vi "RX ADU.vi"(8 "error in (no error)":errorcluster, 9 "PDU_req":T1={"Function Code"=1, "Data"=[], "RTU_DataBytes"=0}, 10 "VISA resource in":refnum<visa-resource-name>, 11 "MB_ADU_Serial_ASCII in":refnum<class "MB_ADU_ASCII.lvclass">) -> (0 "error out":errorcluster, 1 "PDU_resp":T1={"Function Code"=1, "Data"=[], "RTU_DataBytes"=0}, 2 "VISA resource out":refnum<visa-resource-name>, 3 "MB_ADU_Serial_ASCII out":refnum<class "MB_ADU_ASCII.lvclass">)   [LabVIEW 2016, in "MB Master.lvlib" / "MB_ADU_ASCII.lvclass"]
doc: "Defines the receive procedure for a Modbus ASCII ADU. The received PDU is written to PDU_resp."
uses:
  MB_ADU_ASCII.lvclass
  C:/Users/illogicdev/Desktop/IGUS/20190906-1xdryveD1+LABview+ModbusTCP(Gateway)/IgusPositioningSystem Folder/Modules/Libraries/Modbus-Master/MB_ADU/MB_ADU.lvclass
  MB_PDU/MB_PDU_Cluster.ctl
  MB_ADU/MB_ADU.lvclass/MB_ADU.ctl
  MB_ADU/Write RX Data.vi
  MB_ADU/Write RX Timestamp.vi
  MB_ADU/Read Slave ID.vi
  MB Master.lvlib
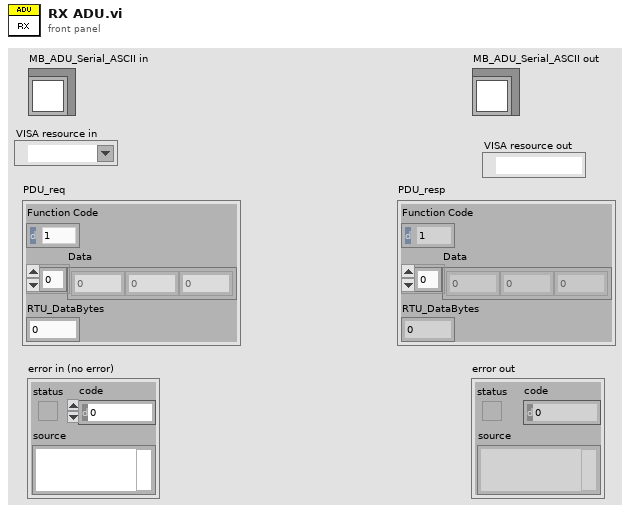
[diagram p1: front panel]
types:
  T1 = typedef "MB Master.lvlib/MB_PDU_Cluster.ctl" = cluster{"Function Code":u8, "Data":u8[], "RTU_DataBytes":i32}
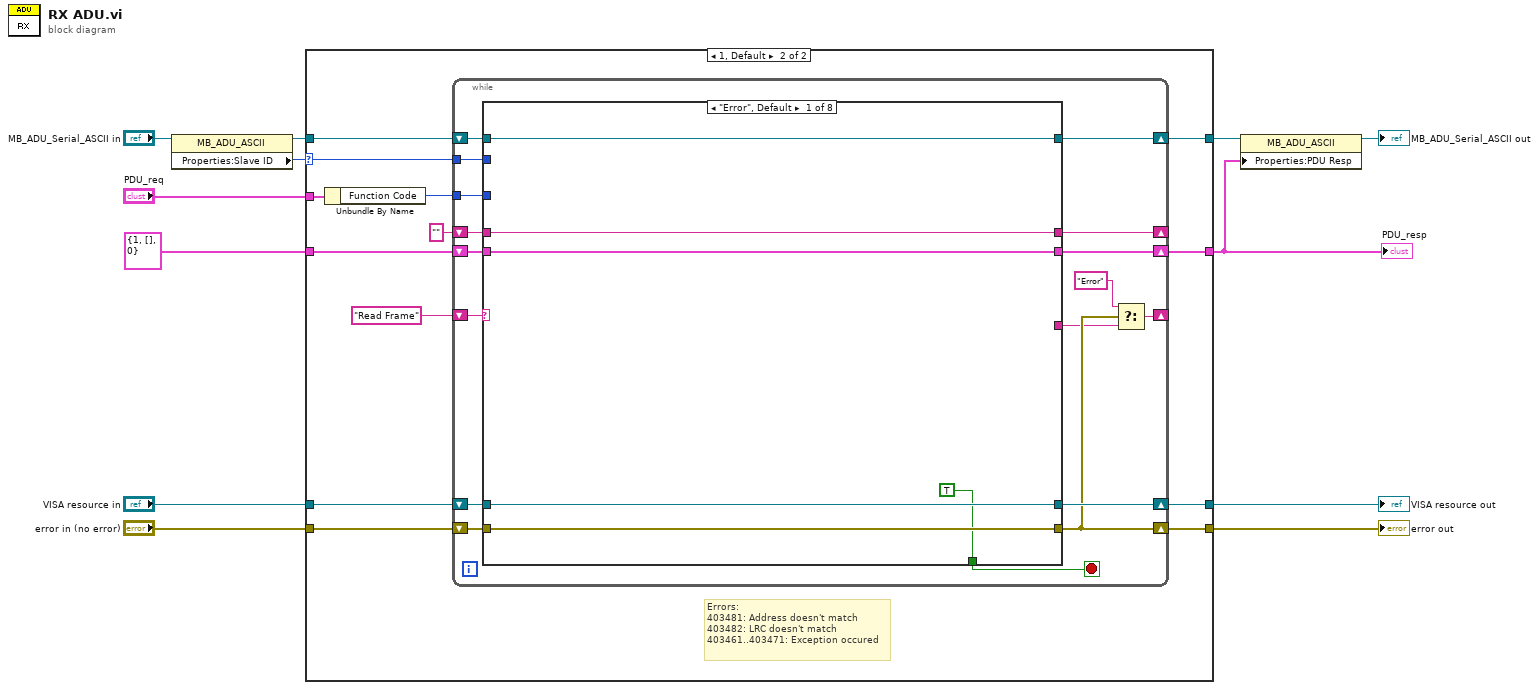
[diagram p0: block diagram]
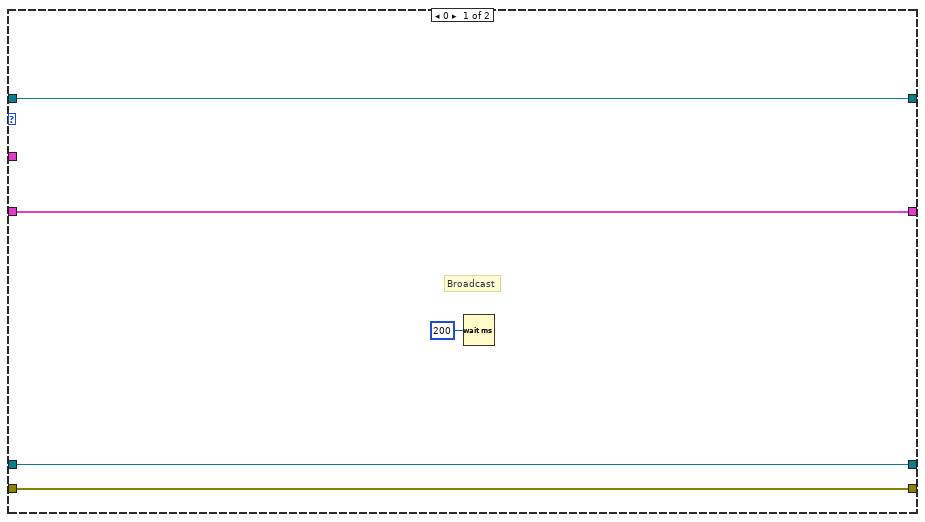
[diagram p2: hidden frame]
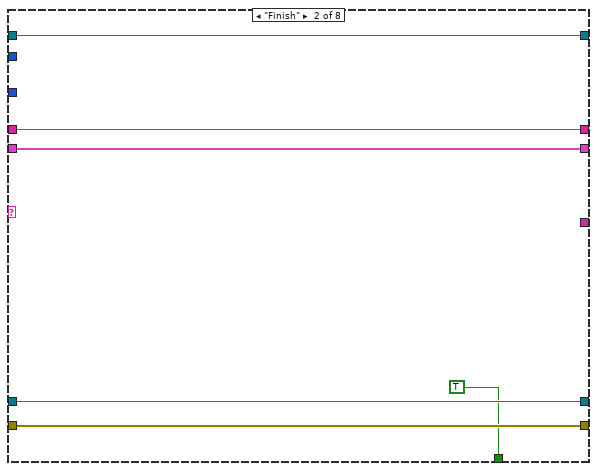
[diagram p3: hidden frame]
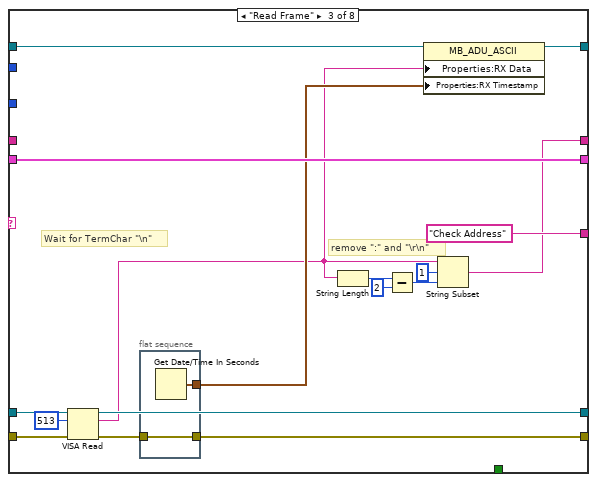
[diagram p4: hidden frame]
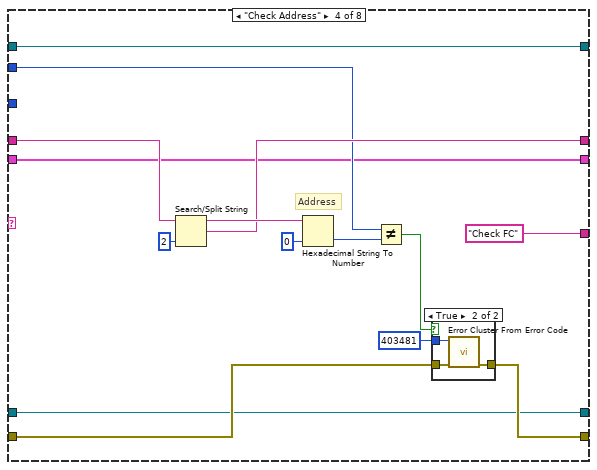
[diagram p5: hidden frame]
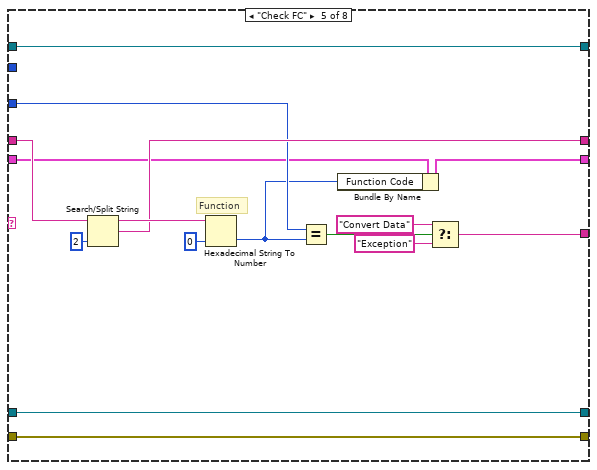
[diagram p7: hidden frame]
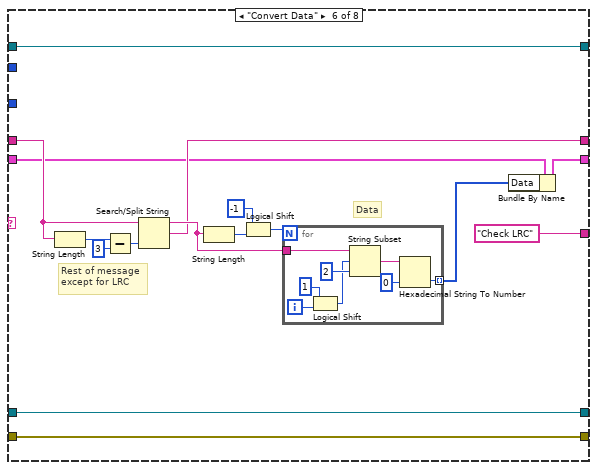
[diagram p8: hidden frame]
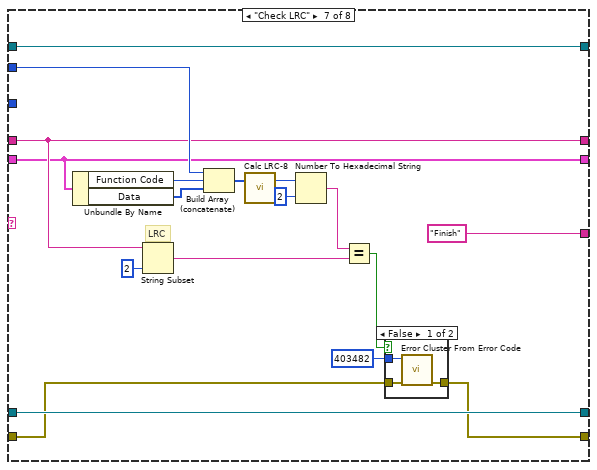
[diagram p9: hidden frame]
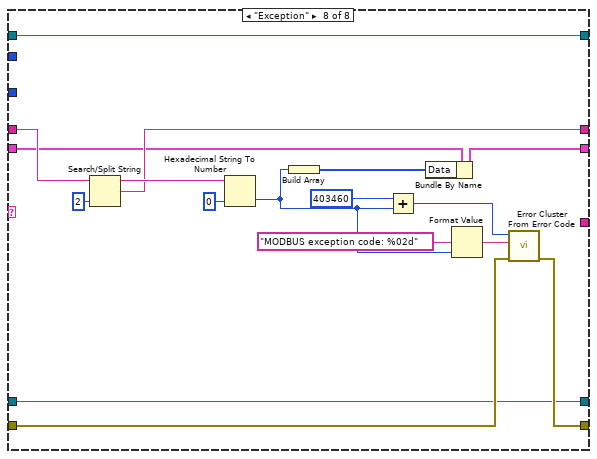
[diagram p11: hidden frame]
diagram:
  n1 = property class="MB_ADU_ASCII"(reference="MB_ADU_Serial_ASCII in") -> (reference out=w7:refnum<class "MB_ADU_ASCII.lvclass">, "Properties:Slave ID"=w6:u8)  [unwired: 1 in, 1 out]
  n2 = case shown="1, Default" w6 {
    selector: w6 -> [_ w20]
    tunnel: "VISA resource in" -> [w15 w30]
    tunnel: "error in (no error)" -> [w14 w29]
    tunnel: T1 {"Function Code"=1, "Data"=[], "RTU_DataBytes"=0} ("PDU_resp") -> [w16 w28]
    tunnel: [w15 w27] -> w9
    tunnel: [w14 w26] -> w8
    tunnel: [w16 w23] -> w1
    tunnel: w7 -> [w17 w22]
    tunnel: [w17 w21] -> w3
    tunnel: "PDU_req" -> [_ w19]
    frame 0 {
      # "Broadcast"
      n3 = Wait (ms)(milliseconds to wait=u32 200) -> ()  [unwired: 1 out]
    }
    frame 1, Default {
      # "Errors:\n403481: Address doesn't match\n403482: LRC doesn't match\n403461..403471: Exception occured"
      n4 = Unbundle By Name(w19) -> ("Function Code"=w18:u8)
      n5 = while {
        shift-right: [w44] -> w27
        shift-left: w30 -> [w47]
        shift-right: [w42] -> w26
        shift-left: w29 -> [w46]
        shift-right: [w43] -> w23
        shift-left: w28 -> [w45]
        shift-right: [w39] -> _
        shift-left: "Read Frame" -> [w36]
        shift-right: [w38] -> _
        shift-left: "" ("read buffer") -> [w37]
        tunnel: w20 -> [w34]
        tunnel: w18 -> [w33]
        shift-right: [w31] -> w21
        shift-left: w22 -> [w32]
        stop <- w35 stop-if-true
        n6 = case shown="\"Error\", Default" w36 {
          tunnel: w47 -> [w52 w58 w75 w81 w103 w123 w147 w164]
          tunnel: w46 -> [w53 w59 w74 w85 w102 w124 w143 w166]
          tunnel: w45 -> [w49 w55 w71 w82 w100 w116 w138 w162]
          tunnel: [w52 w58 w73 w81 w103 w123 w147 w164] -> w44
          tunnel: [w53 w59 w64 w84 w102 w124 w144 w165] -> w42
          tunnel: [w49 w55 w71 w82 w99 w115 w138 w160] -> w43
          tunnel: [_ _ "Check Address" "Check FC" w104 "Check LRC" ("f") "Finish" ("f") _] -> w40
          tunnel: [w50 w56 w69 w89 w110 w117 w150 w168] -> w38
          tunnel: w37 -> [w50 w56 _ w90 w109 w126 w150 w171]
          tunnel: [TRUE TRUE _ _ _ _ _ _] -> w35
          tunnel: w34 -> [_ _ _ w88 _ _ w155 _]
          tunnel: w33 -> [_ _ _ _ w108 _ _ _]
          tunnel: w32 -> [w48 w54 w68 w79 w101 w122 w141 w163]
          tunnel: [w48 w54 w67 w79 w101 w122 w141 w163] -> w31
          frame "Error", Default {
          }
          frame "Finish" {
          }
          frame "Read Frame" {
            # "remove \":\" and \"\\r\\n\""
            # "Wait for TermChar \"\\n\""
            n7 = VISA Read(VISA resource name=w75, byte count=u32 513, error in (no error)=w74) -> (VISA resource name out=w73:refnum<visa-resource-name>, read buffer=w63:string, error out=w65:errorcluster)  [unwired: 1 out]
            n8 = flat-sequence {
              tunnel: [w78] -> w66
              tunnel: w65 -> [w77]
              tunnel: [w77] -> w64
              frame #0 {
                n9 = Get Date/Time In Seconds() -> (seconds since 1Jan1904=w78:timestamp)
              }
            }
            n10 = String Length(string=w63) -> (length=w62:i32)
            n11 = Subtract(x=w62, y=2) -> (x-y=w60:i32)
            n12 = property class="MB_ADU_ASCII"(reference=w68, "Properties:RX Data"=w63, "Properties:RX Timestamp"=w66) -> (reference out=w67:refnum<class "MB_ADU_ASCII.lvclass">)  [unwired: 1 in, 1 out]
            n13 = String Subset(string=w63, offset (0)=1, length (rest)=w60) -> (substring=w69:string)
          }
          frame "Check Address" {
            # "Address"
            n14 = Search/Split String(string=w90, offset (0)=2) -> (substring before match=w91:string, match + rest of string=w89:string)  [unwired: 1 in, 1 out]
            n15 = Hexadecimal String To Number(string=w91, default (0uL)=u8 0) -> (number=w87:u8)  [unwired: 1 in, 1 out]
            n16 = Not Equal?(x=w88, y=w87) -> (x != y?=w83:bool)
            n17 = case shown="True" w83 {
              tunnel: [w94 w96] -> w84
              tunnel: w85 -> [w94 w97]
              tunnel: 403481 ("error code (0)") -> [_ w95]
              frame False {
              }
              frame True {
                n18 = call <vilib>:"Error Cluster From Error Code.vi"("error in (no error)"=w97, "error code (0)"=w95) -> ("error out"=w96:errorcluster)  [unwired: 7 in]
              }
            }
          }
          frame "Check FC" {
            # "Function"
            n19 = Search/Split String(string=w109, offset (0)=2) -> (substring before match=w111:string, match + rest of string=w110:string)  [unwired: 1 in, 1 out]
            n20 = Hexadecimal String To Number(string=w111, default (0uL)=u8 0) -> (number=w98:u8)  [unwired: 1 in, 1 out]
            n21 = Equal?(x=w108, y=w98) -> (x = y?=w107:bool)
            n22 = Bundle By Name(cluster=w100, "Function Code"=w98) -> (w99:T1)
            n23 = Select(t="Convert Data", s=w107, f="Exception") -> (s? t:f=w104:string)
          }
          frame "Convert Data" {
            # "Data"
            # "Rest of message\nexcept for LRC"
            n24 = String Length(string=w126) -> (length=w128:i32)
            n25 = Subtract(x=w128, y=3) -> (x-y=w127:i32)
            n26 = Search/Split String(string=w126, offset (0)=w127) -> (substring before match=w118:string, match + rest of string=w117:string)  [unwired: 1 in, 1 out]
            n27 = String Length(string=w118) -> (length=w121:i32)
            n28 = Logical Shift(y=i16 -1, x=w121) -> (x << y=w119:i32)
            n29 = for {
              N: w119 -> [_]
              tunnel: [w136] -> w114 mode=indexing
              tunnel: w118 -> [w135]
              i -> [w132]
              n30 = Logical Shift(y=i16 1, x=w132) -> (x << y=w130:i32)
              n31 = String Subset(string=w135, offset (0)=w130, length (rest)=2 ("y")) -> (substring=w133:string)
              n32 = Hexadecimal String To Number(string=w133, default (0uL)=u8 0) -> (number=w136:u8)  [unwired: 1 in, 1 out]
            }
            n33 = Bundle By Name(cluster=w116, "Data"=w114) -> (w115:T1)
          }
          frame "Check LRC" {
            # "LRC"
            n34 = Unbundle By Name(w138) -> ("Function Code"=w140:u8, "Data"=w139:u8[])
            n35 = String Subset(string=w150, length (rest)=2 ("length (rest)")) -> (substring=w148:string)  [unwired: 1 in]
            n36 = Build Array (concatenate)(w155, w140, w139) -> (w154:u8[])
            n37 = call "Calc LRC-8.vi"("Frame in"=w154) -> ("LRC-8"=w153:u8)  [unwired: 2 in]
            n38 = Number To Hexadecimal String(1:i16 2 ("width (-)"), 2:w153) -> (0:w151:string)
            n39 = Equal?(x=w151, y=w148) -> (x = y?=w145:bool)
            n40 = case shown="False" w145 {
              tunnel: [w157 w159] -> w144
              tunnel: w143 -> [w158 w159]
              tunnel: 403482 ("error code (0)") -> [w156 _]
              frame False {
                n41 = call <vilib>:"Error Cluster From Error Code.vi"("error in (no error)"=w158, "error code (0)"=w156) -> ("error out"=w157:errorcluster)  [unwired: 7 in]
              }
              frame True {
              }
            }
          }
          frame "Exception" {
            n42 = Search/Split String(string=w171, offset (0)=2) -> (substring before match=w170:string, match + rest of string=w168:string)  [unwired: 1 in, 1 out]
            n43 = Hexadecimal String To Number(string=w170, default (0uL)=u8 0) -> (number=w167:u8)  [unwired: 1 in, 1 out]
            n44 = Build Array(w167) -> (w161:u8[])
            n45 = Add(x=403460 ("error code (0)"), y=w167) -> (x+y=w173:i32)
            n46 = Bundle By Name(cluster=w162, "Data"=w161) -> (w160:T1)
            n47 = Format Value(format string="MODBUS exception code: %02d", value (0)=w167) -> (output string=w175:string)  [unwired: 1 in]
            n48 = call <vilib>:"Error Cluster From Error Code.vi"("error in (no error)"=w166, "error message (\"\")"=w175, "error code (0)"=w173) -> ("error out"=w165:errorcluster)  [unwired: 6 in]
          }
        }
        n49 = Select(t="Error", s=w42, f=w40) -> (s? t:f=w39:string)
      }
    }
  }
  "error out" <- w8
  "VISA resource out" <- w9
  "PDU_resp" <- w1
  n50 = property class="MB_ADU_ASCII"(reference=w3, "Properties:PDU Resp"=w1) -> (reference out=→"MB_ADU_Serial_ASCII out":refnum<class "MB_ADU_ASCII.lvclass">)  [unwired: 1 in, 1 out]
